vi "initializeStyle.vi"(8 "error in (no error)":errorcluster, 10 "Style":refnum<class "Style.lvclass">, 11 "xwpfRun.Header1 in":refnum<class "xwpfRun.Header1.lvclass">) -> (0 "error out":errorcluster, 3 "xwpfRun.Header1 out":refnum<class "xwpfRun.Header1.lvclass">)   [LabVIEW 2017, in "Word_Specific.lvlib" / "xwpfRun.Header1.lvclass"]
uses:
  xwpfRun.Header1.lvclass
  Styles/Style/Style.lvclass
  Styles/Heading 1/Heading 1.lvclass
  C:/Users/Neo/Desktop/Dev_Tools_BR/LabVIEW_NPOI/src/Styles/Style/Style.lvclass
  xwpfRun/xwpfRun.lvclass
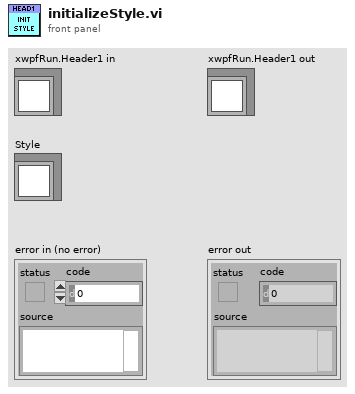
[diagram p1: front panel]
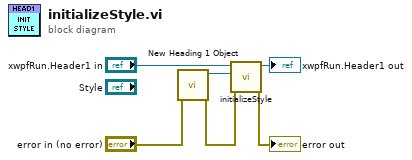
[diagram p0: block diagram]
diagram:
  n1 = call "New Heading 1 Object.vi"("error in (no error)"="error in (no error)") -> ("error out"=w1:errorcluster, "Heading 1 out"=w3:refnum<class "Heading 1.lvclass">)  [unwired: 9 in]
  n2 = call-parent "initializeStyle.vi"("error in (no error)"=w1, "Style"=w3, "xwpfRun in"="xwpfRun.Header1 in") -> ("error out"=→"error out":errorcluster, "xwpfRun out"=→"xwpfRun.Header1 out":refnum<class "xwpfRun.Header1.lvclass">)  [unwired: 7 in]
